vi "ObtainQueue.vi"(11 "queueName":string) -> (3 "queue":string)   [LabVIEW 2011]
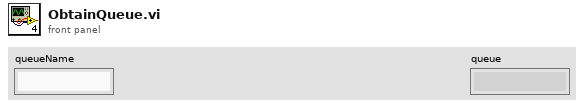
[diagram p1: front panel]
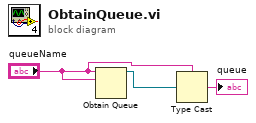
[diagram p0: block diagram]
diagram:
  n1 = Obtain Queue(name (unnamed)="queueName", element data type="queueName") -> (queue out=w3:refnum<queue>)  [unwired: 3 in, 2 out]
  n2 = Type Cast(type="queueName", x=w3) -> (*(type *) &x=→"queue":string)
